vi "item name.vi"() -> ()   [LabVIEW 2020]
panel:
  out "Item Names":string[][](array[string])
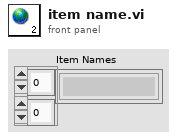
[diagram p1: front panel]
diagram:
